vi "compet.vi"() -> ()   [LabVIEW 2020]
panel:
  out "min index(es)":i32
  out "Array 2":dbl[](array[numeric])=[0.15, 0.89, 0.7, 0.05, 0.324, 0.2345, 0.4875, 0.075, 0.968, -0.6153]
  out "min value":dbl
  out "output array":dbl[](array[numeric])
  in  "Numeric":dbl format="%#_13g"
  out "Array":dbl[](array[numeric])
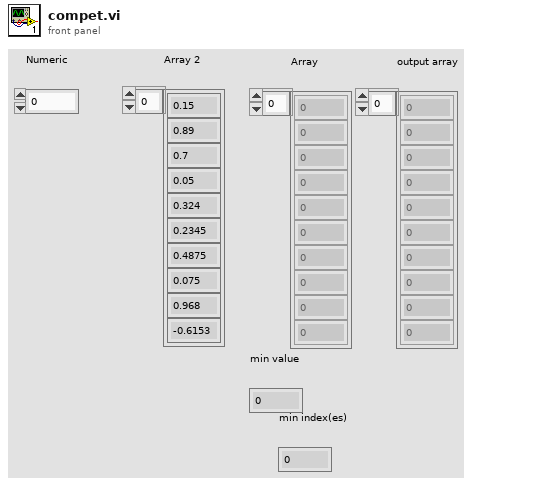
[diagram p1: front panel]
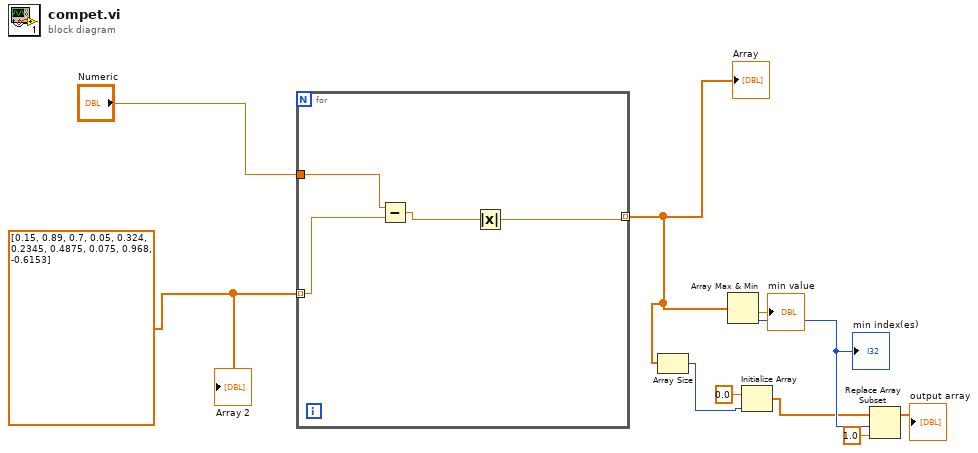
[diagram p0: block diagram]
diagram:
  w10 = dbl[] [0.15, 0.89, 0.7, 0.05, 0.324, 0.2345, 0.4875, 0.075, 0.968, -0.6153]
  n1 = for {
    tunnel: w10 -> [w13] mode=indexing
    tunnel: "Numeric" -> [w14]
    tunnel: [w11] -> w7 mode=indexing
    n2 = Subtract(x=w14, y=w13) -> (x-y=w12:dbl)
    n3 = Absolute Value(x=w12) -> (abs(x)=w11:dbl)
  }
  "Array" <- w7
  n4 = Array Size(array=w7) -> (size(s)=w6:i32)
  n5 = Array Max & Min(array=w7) -> (min value=→"min value":dbl, min index (indices)=w5:i32)  [unwired: 2 out]
  "min index(es)" <- w5
  n6 = Initialize Array(0.0 ("element"), w6) -> (w4:dbl[])
  n7 = Replace Array Subset(array=w4, new element=1.0 ("new element/subarray"), index=w5) -> (→"output array":dbl[])
  "Array 2" <- w10
